vi "Read_Instr.vi"(8 "error in (no error)":errorcluster caption="entrée d'erreur (pas d'erreur)", 11 "Class Instrument Multimeter en entrée":refnum<class "Class Instrument Schielding_Box.lvclass">) -> (0 "error out":errorcluster caption="sortie d'erreur", 3 "Class Instrument Multimeter en sortie":refnum<class "Class Instrument Schielding_Box.lvclass">)   [LabVIEW 2020, in "Library Instrument & Equipement.lvlib" / "Library Instruments.lvlib" / "Class Instrument Schielding_Box.lvclass"]
uses:
  Class Instrument Schielding_Box.lvclass
  Class Instrument Schielding_Box.lvclass/Class Instrument Schielding_Box.ctl
  Instrument (Default)/Class Instrument (Default).lvclass
  Shielding box/Class Shielding box (Default)/Class Shielding_ Box (Default).lvclass
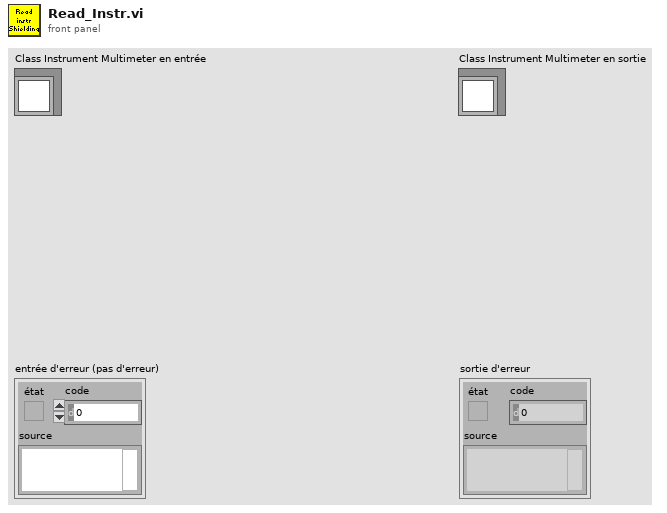
[diagram p1: front panel]
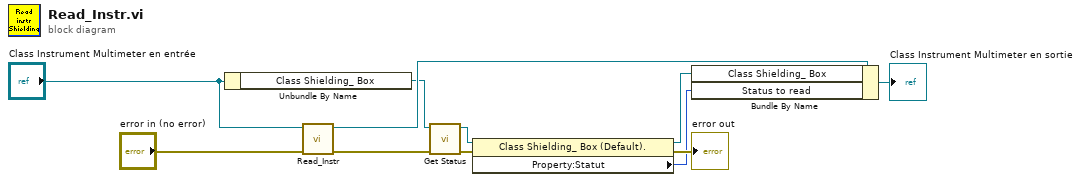
[diagram p0: block diagram]
diagram:
  n1 = Unbundle By Name("Class Instrument Multimeter en entrée") -> ("Class Shielding_ Box"=w5:refnum<class "Class Shielding_ Box (Default).lvclass">)
  n2 = call-parent "Read_Instr.vi"("error in (no error)"="error in (no error)", "Class Instrument (Default) en entrée"="Class Instrument Multimeter en entrée") -> ("error out"=w4:errorcluster, "Class Instrument (Default) en sortie"=w6:refnum<class "Class Instrument Schielding_Box.lvclass">)  [unwired: 8 in]
  n3 = call-dynamic "Get Status.vi"("error in (no error)"=w4, "Class Shielding_ Box en entrée"=w5) -> ("error out"=w3:errorcluster, "Class Shielding_ Box en sortie"=w2:refnum<class "Class Shielding_ Box (Default).lvclass">)  [unwired: 8 in]
  n4 = property class="Class Shielding_ Box (Default)."(reference=w2, error in=w3) -> (reference out=w8:refnum<class "Class Shielding_ Box (Default).lvclass">, error out=→"error out":errorcluster, "Property:Statut"=w1:enum16{"Erreur", "Close", "Open"})
  n5 = Bundle By Name(cluster=w6, "Class Shielding_ Box"=w8, "Status to read"=w1) -> (→"Class Instrument Multimeter en sortie":refnum<class "Class Instrument Schielding_Box.lvclass">)
